vi "OAT AC DC Separation (N Channels).vi"(0 "even-angle signals":cluster{"r0":dbl, "dr":dbl, "Y":dbl[]}[](array[cluster]) {"r0" format="%.2p"; "dr" format="%.2p"; "Y" format="%.2f"}, 1 "even-angle channel info":T2[](array[typedef]) {"channel info"."pregain" format="%.2f"; "channel info"."weighting filter" items=["Linear", "A-weighting", "B-weighting", "C-weighting", "ITU-R 468-4", "Dolby", "CCITT", "C-message", "Wb", "Wc", "Wd", "We", "Wf", "Wh", "Wj", "Wk", "Wm", "AES17 20 kHz lowpass", "AES17 40 kHz lowpass", "AES17 20 kHz highpass", "AES17 40 kHz highpass"]; "channel info"."dB reference" format="%^.1e"; "channel info"."engineering units" items=["custom..."=0, "V"=1, "A"=21, "C"=30, "pC"=31, "s"=32, "-"=29, "Pa"=2, "N"=20, "g"=3, "m/s^2"=4, "m/s"=5, "m"=6, "mm/s"=12, "mm"=13, "micron/s"=14, "micron"=15, "in/s^2"=7, "in/s"=8, "in"=9, "mil/s"=10, "mil"=11, "rad/s^2"=16, "rad/s"=17, "rad"=18, "deg/s^2"=26, "deg/s"=27, "deg"=28, "RPM"=22, "cycle/s^2"=23, "Hz"=24, "cycle"=25, "strain"=19]; "channel info"."sensor sensitivity" format="%#_5f"}, 2 "revolution number (1)":dbl=1.0 min=0.0, 3 "position info":T1, 5 "error in (no error)":errorcluster, 8 "reset? (F)":bool) -> (12 "unit labels":string[](array[string]), 14 "even-angle AC signals":cluster{"r0":dbl, "dr":dbl, "Y":dbl[]}[](array[cluster]) {"r0" format="%.2p"; "dr" format="%.2p"; "Y" format="%.2f"}, 15 "dup even-angle channel info":T2[](array[typedef]) {"channel info"."pregain" format="%.2f"; "channel info"."weighting filter" items=["Linear", "A-weighting", "B-weighting", "C-weighting", "ITU-R 468-4", "Dolby", "CCITT", "C-message", "Wb", "Wc", "Wd", "We", "Wf", "Wh", "Wj", "Wk", "Wm", "AES17 20 kHz lowpass", "AES17 40 kHz lowpass", "AES17 20 kHz highpass", "AES17 40 kHz highpass"]; "channel info"."dB reference" format="%^.1e"; "channel info"."engineering units" items=["custom..."=0, "V"=1, "A"=21, "C"=30, "pC"=31, "s"=32, "-"=29, "Pa"=2, "N"=20, "g"=3, "m/s^2"=4, "m/s"=5, "m"=6, "mm/s"=12, "mm"=13, "micron/s"=14, "micron"=15, "in/s^2"=7, "in/s"=8, "in"=9, "mil/s"=10, "mil"=11, "rad/s^2"=16, "rad/s"=17, "rad"=18, "deg/s^2"=26, "deg/s"=27, "deg"=28, "RPM"=22, "cycle/s^2"=23, "Hz"=24, "cycle"=25, "strain"=19]; "channel info"."sensor sensitivity" format="%#_5f"}, 16 "even-angle DC signals":cluster{"r0":dbl, "dr":dbl, "Y":dbl[]}[](array[cluster]) {"r0" format="%.2p"; "dr" format="%.2p"; "Y" format="%.2f"}, 17 "position info out":T1, 19 "error out":errorcluster)   [LabVIEW 2017, in "SoundVib_OAUtility.lvlib"]
doc: "Separates and returns the AC and DC levels of the <B>even-angle signal</B> by continuously removing the DC values from the signal. This VI calculates the DC values over the interval specified by the <B>revolution number</B>. Wire data to the <B>even-angle signal</B> input to determine the polymorphic instance to use or manually select the instance."
uses:
  <vilib>/addons/Sound and Vibration/Order Analysis/Utility/SoundVib_OAUtility.lvlib
  <vilib>/addons/_NISVFA/_Shared subVIs/Controls/svc_Resampled Channel Info.ctl
  <vilib>/addons/_NISVFA/_Shared subVIs/Controls/svc_Channel Info.ctl
  <vilib>/addons/_NISVFA/_Shared subVIs/Controls/svc_Engineering Units Text Ring.ctl
  <vilib>/addons/_NISVFA/_Shared subVIs/Controls/svc_Weighting Filter Text Ring.ctl
  <vilib>/addons/Sound and Vibration/Order Analysis/Misc/OAT Position Info.ctl
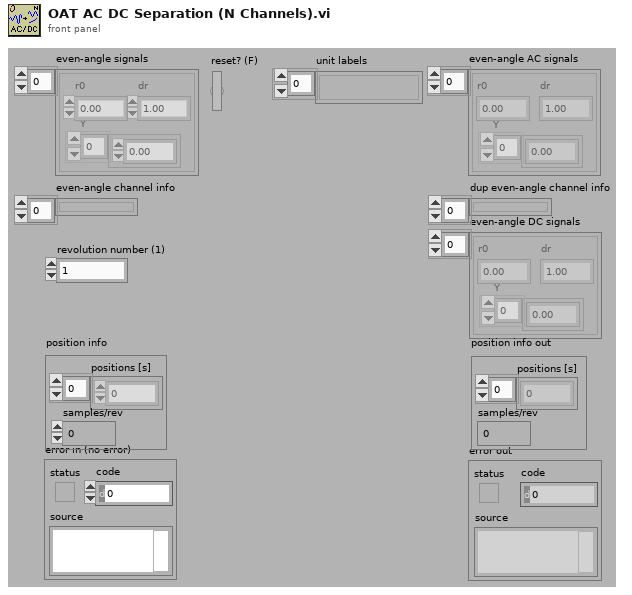
[diagram p1: front panel]
types:
  T1 = typedef "OAT Position Info.ctl" = cluster{"positions [s]":dbl[], "samples/rev":dbl}
  T2 = typedef "svc_Resampled Channel Info.ctl" = cluster{"channel name":string, "description":string, " channel info":T3}
  T3 = typedef "svc_Channel Info.ctl" = cluster{"sensor sensitivity":dbl, "engineering units":T4, "dB reference":dbl, "custom label":string, "weighting filter":T5, "pregain":dbl}
  T4 = typedef "svc_Engineering Units Text Ring.ctl" = u16
  T5 = typedef "svc_Weighting Filter Text Ring.ctl" = u16
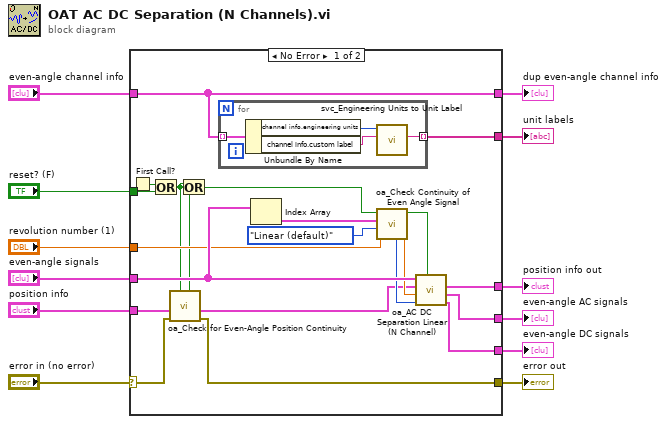
[diagram p0: block diagram]
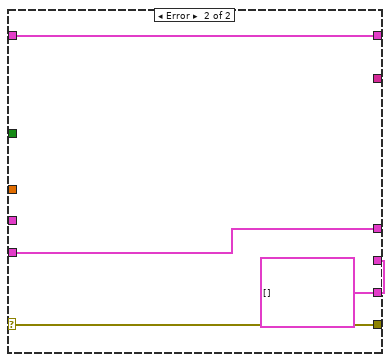
[diagram p2: hidden frame]
diagram:
  n1 = case shown="No Error" "error in (no error)" {
    selector: "error in (no error)" -> [w14 w41]
    tunnel: [w13 w41] -> w11
    tunnel: [w22 w38] -> w9
    tunnel: "even-angle channel info" -> [w22 w38]
    tunnel: "reset? (F)" -> [w33 _]
    tunnel: "even-angle signals" -> [w30 _]
    tunnel: [w28 w40] -> w6
    tunnel: [w27 w40] -> w5
    tunnel: "revolution number (1)" -> [w25 _]
    tunnel: [w21 _] -> w3
    tunnel: "position info" -> [w20 w39]
    tunnel: [w19 w39] -> w1
    frame No Error {
      n2 = First Call?() -> (First Call?: T/F=w32:bool)
      n3 = Or(x=w32, y=w33) -> (x .or. y?=w17:bool)
      n4 = call <vilib>:"oa_Check for Even-Angle Position Continuity.vi"("reset in"=w17, "error in (no error)"=w14, "even-angle position info"=w20) -> ("error out"=w13:errorcluster, "even-angle position info dup"=w18:T1, "position not continuous"=w15:bool)  [unwired: 6 in]
      n5 = Or(x=w17, y=w15) -> (x .or. y?=w16:bool)
      n6 = for {
        tunnel: w22 -> [w37] mode=indexing
        tunnel: [w36] -> w21 mode=indexing
        n7 = Unbundle By Name(w37) -> ("channel info.engineering units"=w35:T4, "channel info.custom label"=w34:string)
        n8 = call <vilib>:"svc_Engineering Units to Unit Label.vi"("custom label"=w34, "engineering units"=w35) -> ("unit label"=w36:string)  [unwired: 8 in, 1 out]
      }
      n9 = Index Array(array=w30) -> (element=w31:cluster{"r0":dbl, "dr":dbl, "Y":dbl[]})  [unwired: 1 in]
      n10 = call <vilib>:"oa_Check Continuity of Even Angle Signal.vi"("averaging revolution (1)"=w25, "averaging type"=enum16{"Linear (default)", "Exponential", "Mix"}."Linear (default)", "even angle signal"=w31, "reset?(F)"=w16) -> ("dul averaging revolution"=w23:dbl, "reset out"=w29:bool, "points/rev"=w26:u32)  [unwired: 3 in, 2 out]
      n11 = call <vilib>:"oa_AC DC Separation Linear (N Channel).vi"("reset? (F)"=w29, "points/rev"=w26, "averaging revolution (1)"=w23, "position info"=w18, "even angle signals"=w30) -> ("DC even angle signals"=w27:cluster{"r0":dbl, "dr":dbl, "Y":dbl[]}[], "AC even angle signals"=w28:cluster{"r0":dbl, "dr":dbl, "Y":dbl[]}[], "position info out"=w19:T1)  [unwired: 3 in, 1 out]
    }
    frame Error {
      w40 = cluster{"r0":dbl, "dr":dbl, "Y":dbl[]}[] []
    }
  }
  "error out" <- w11
  "even-angle DC signals" <- w5
  "even-angle AC signals" <- w6
  "dup even-angle channel info" <- w9
  "position info out" <- w1
  "unit labels" <- w3
